vi "CLEAR ARRAY.vi"(9 "Array in":string[](array[string])) -> (1 "Array out":string[](array[string]))   [LabVIEW 2017]
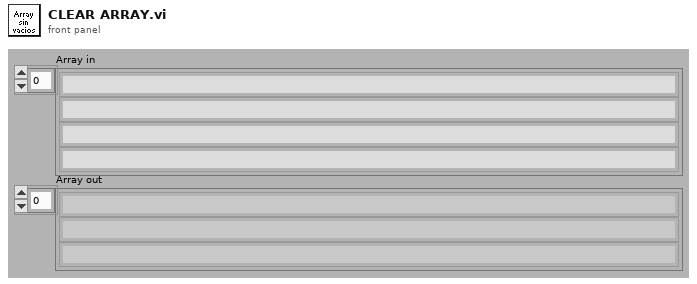
[diagram p1: front panel]
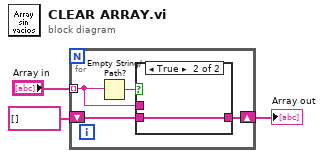
[diagram p0: block diagram]
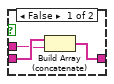
[diagram p2: hidden frame]
diagram:
  n1 = for {
    tunnel: "Array in" -> [w5] mode=indexing
    shift-right: [w6] -> w1
    shift-left: string[] [] -> [w7]
    n2 = Empty String/Path?(string/path=w5) -> (empty?=w4:bool)
    n3 = case shown="True" w4 {
      tunnel: w7 -> [w10 w11]
      tunnel: w5 -> [w9 _]
      tunnel: [w8 w11] -> w6
      frame False {
        n4 = Build Array (concatenate)(w10, w9) -> (w8:string[])
      }
      frame True {
      }
    }
  }
  "Array out" <- w1
